vi "StringToNode(viaString).vi"(0 "Tree DVR in":refnum<data-value>, 1 "String value in":string, 3 "error in (no error)":errorcluster, 4 "NodePath":string) -> (5 "Tree DVR out":refnum<data-value>, 6 "TreeNode DVR out":refnum<data-value>, 7 "error out":errorcluster)   [LabVIEW 2013]
uses:
  <vilib>/MDSplus/Classes/Tree_Class/Tree.lvclass
  <vilib>/MDSplus/Classes/Data_Class/TreeNode_Class/TreeNode.lvclass
  <vilib>/MDSplus/Library/MDSplus.lvlib
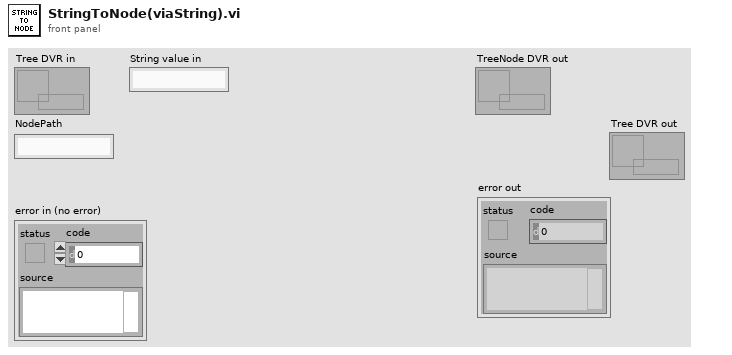
[diagram p1: front panel]
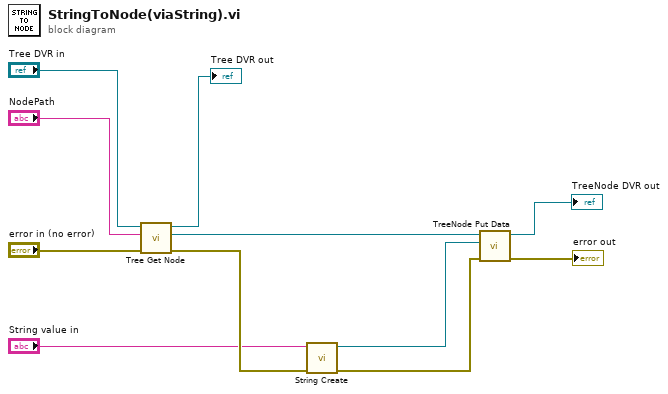
[diagram p0: block diagram]
diagram:
  n1 = call <vilib>:"Tree Get Node.vi"("error in (no error)"="error in (no error)", "Path"="NodePath", "Tree DVR in"="Tree DVR in") -> ("error out"=w2:errorcluster, "Node out"=w11:refnum<data-value>, "Tree DVR out"=→"Tree DVR out":refnum<data-value>)  [unwired: 6 in]
  n2 = call <vilib>:"String Create.vi"("error in (no error)"=w2, "String value in"="String value in") -> ("error out"=w3:errorcluster, "String DVR out"=w4:refnum<data-value>)  [unwired: 8 in]
  n3 = call <vilib>:"TreeNode Put Data.vi"("error in (no error)"=w3, "Data"=w4, "TreeNode DVR in"=w11) -> ("error out"=→"error out":errorcluster, "TreeNode DVR out"=→"TreeNode DVR out":refnum<data-value>)  [unwired: 7 in]
